vi "Log Message.vi"(6 "Log Category (application)":string="application", 8 "error in (no error)":errorcluster, 10 "Log File Name (see Default Log File.vi)":path, 11 "Message to Log":string) -> (0 "error out":errorcluster)   [LabVIEW 2020, in "RxnRover.lvlib" / "logging.lvlib"]
doc: "Logs the given message to a log file in the Rxn Rover log directory. If no log file is provided, the default log file name is used. See Default Log File.vi for more details about the form of the default log file name."
uses:
  logging.lvlib
  File IO/Project Locations/Project Locations.lvlib
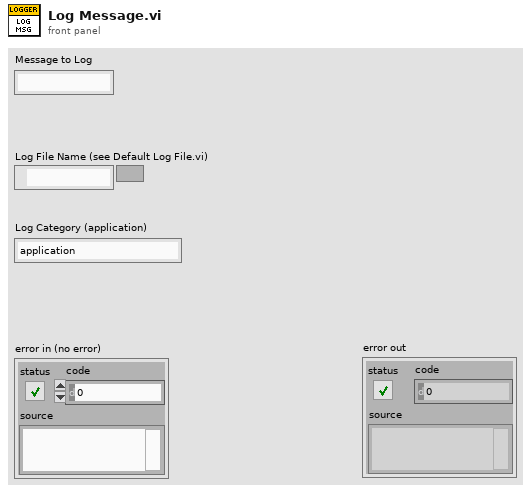
[diagram p1: front panel]
types:
  T1 = enum16{"open", "replace", "create", "open or create", "replace or create", "replace or create with confirmation"}
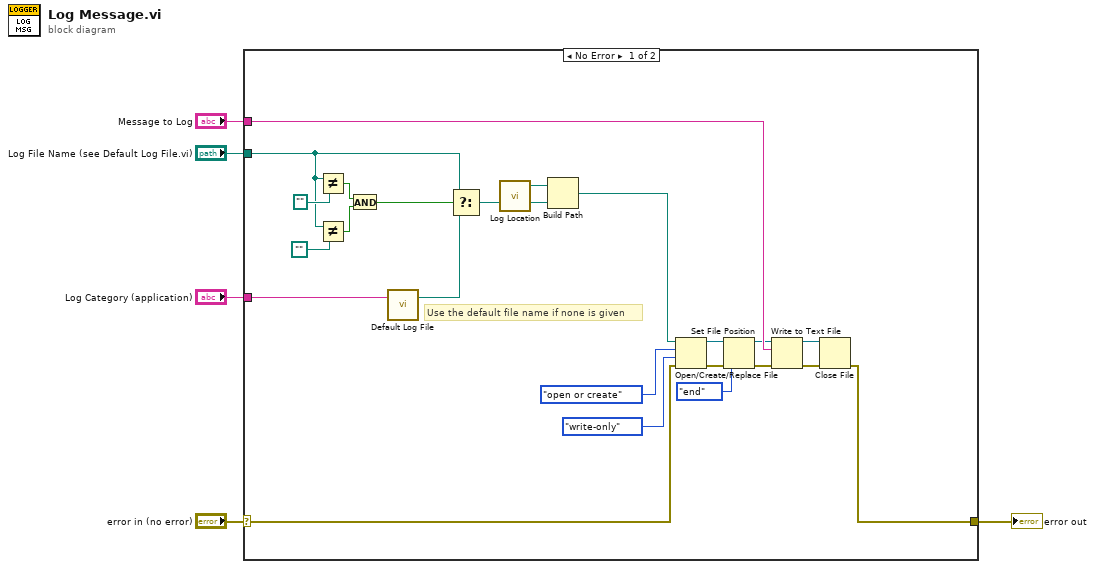
[diagram p0: block diagram]
diagram:
  n1 = case shown="No Error" "error in (no error)" {
    selector: "error in (no error)" -> [w13 w29]
    tunnel: [w12 w29] -> w4
    tunnel: "Log File Name (see Default Log File.vi)" -> [w22 _]
    tunnel: "Message to Log" -> [w19 _]
    tunnel: "Log Category (application)" -> [w6 _]
    frame No Error {
      # "Use the default file name if none is given"
      n2 = Not Equal?(x=w22, y=path "") -> (x != y?=w24:bool)
      n3 = Not Equal?(x=w22, y=path "") -> (x != y?=w23:bool)
      n4 = And(x=w24, y=w23) -> (x .and. y?=w21:bool)
      n5 = call "Default Log File.vi"("Log Category (application)"=w6) -> ("Default Log File Name"=w20:path)  [unwired: 2 in]
      n6 = Select(t=w22, s=w21, f=w20) -> (s? t:f=w16:path)
      n7 = call "Log Location.vi"() -> ("Log Location"=w15:path)  [unwired: 2 in]
      n8 = Build Path(base path=w15, name or relative path=w16) -> (appended path=w14:path)
      n9 = Open/Create/Replace File(file path (use dialog)=w14, error in=w13, operation (0:open)=T1."open or create", access (0:read/write)=enum16{"read/write", "read-only", "write-only"}."write-only") -> (refnum out=w9:refnum<file>, error out=w11:errorcluster)  [unwired: 2 in, 1 out]
      n10 = Set File Position(refnum=w9, from (0:start)=enum16{"start", "end", "current"}."end", error in=w11) -> (refnum out=w8:refnum<file>, error out=w10:errorcluster)  [unwired: 1 in]
      n11 = Write to Text File(file (use dialog)=w8, text=w19, error in=w10) -> (refnum out=w27:refnum<file>, error out=w28:errorcluster)  [unwired: 1 in, 1 out]
      n12 = Close File(refnum=w27, error in=w28) -> (error out=w12:errorcluster)  [unwired: 1 out]
    }
    frame Error {
    }
  }
  "error out" <- w4
